vi "Bin Flush Data to Log File.vi"(8 "error in (no error)":errorcluster, 10 "Data Queue":refnum<queue>, 11 "Logging Configuration":T1) -> (0 "error out":errorcluster)   [LabVIEW 2018, in "Logging.lvlib"]
uses:
  Logging.lvlib
  Logging Configuration.ctl
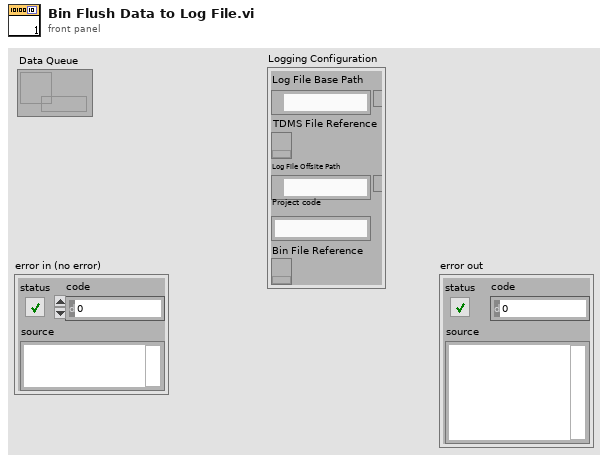
[diagram p1: front panel]
types:
  T1 = typedef "Logging.lvlib/Logging Configuration.ctl" = cluster{"Log File Base Path":path, "TDMS File Reference":refnum<k34>, "Log File Offsite Path":path, "Project code":string, "Bin File Reference":refnum<k34>}
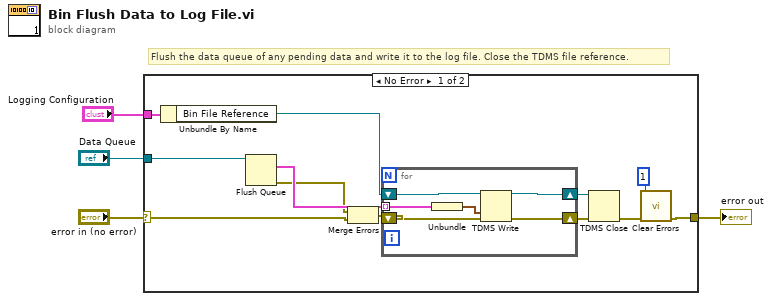
[diagram p0: block diagram]
diagram:
  # "Flush the data queue of any pending data and write it to the log file. Close the TDMS file reference."
  n1 = case shown="No Error" "error in (no error)" {
    selector: "error in (no error)" -> [w15 w23]
    tunnel: "Data Queue" -> [w11 _]
    tunnel: "Logging Configuration" -> [w13 _]
    tunnel: [w6 w23] -> w2
    frame No Error {
      n2 = Unbundle By Name(w13) -> ("Bin File Reference"=w12:refnum<k34>)
      n3 = Flush Queue(queue=w11) -> (remaining elements=w16:cluster{"Array":waveform(dbl)[]}[], error out=w10:errorcluster)  [unwired: 1 in, 1 out]
      n4 = Merge Errors(w10, w15) -> (w14:errorcluster)
      n5 = for {
        shift-right: [w19] -> w8
        shift-left: w12 -> [w20]
        shift-right: [w21] -> w9
        shift-left: w14 -> [w22]
        tunnel: w16 -> [w18] mode=indexing
        n6 = Unbundle(w18) -> ("Array"=w17:waveform(dbl)[])
        n7 = TDMS Write(0:w20, 9:w17, 11:w22) -> (4:w19:refnum<k34>, 15:w21:errorcluster)  [unwired: 3 in, 2 out]
      }
      n8 = TDMS Close(8:w9, 11:w8) -> (0:w7:errorcluster)  [unwired: 1 out]
      n9 = call <vilib>:"Clear Errors.vi"("error in (no error)"=w7, "specific error code to clear (0: all)"=1) -> ("error out"=w6:errorcluster)  [unwired: 4 in, 1 out]
    }
    frame Error {
    }
  }
  "error out" <- w2
